vi "Initialize (No Resource).vi"(11 "error in (no error)":errorcluster) -> (4 "SLSC Local out":refnum<class "SLSC Local.lvclass">, 15 "error out":errorcluster)   [LabVIEW 2015, in "SLSC Local.lvclass"]
uses:
  SLSC Local.lvclass
  SLSC Local.lvclass/SLSC Local.ctl
  <vilib>/SLSC/Initialize Session without Resources.vi
  <vilib>/SLSC/SLSC.lvlib
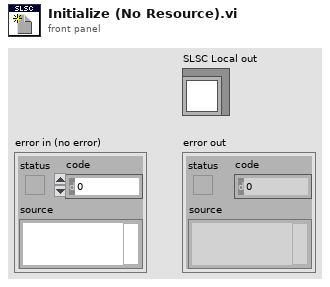
[diagram p1: front panel]
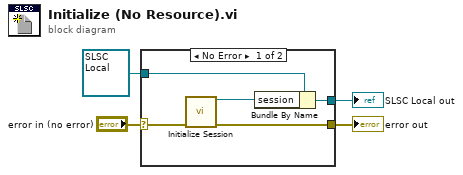
[diagram p0: block diagram]
diagram:
  n1 = case shown="No Error" "error in (no error)" {
    selector: "error in (no error)" -> [w7 w11]
    tunnel: [w6 w11] -> w3
    tunnel: [w8 w10] -> w1
    tunnel: refnum<class "SLSC Local.lvclass"> refnum ("SLSC Local in") -> [w9 w10]
    frame No Error {
      n2 = call-poly <vilib>:"Initialize Session.vi"("error in (no error)"=w7) -> ("session out"=w5:refnum<k21>, "error out"=w6:errorcluster)  [unwired: 13 in]
      n3 = Bundle By Name(cluster=w9, "session"=w5) -> (w8:refnum<class "SLSC Local.lvclass">)
    }
    frame Error {
    }
  }
  "error out" <- w3
  "SLSC Local out" <- w1
